vi "dt.vi"(1 "Locations Peaks":dbl[](array[numeric])) -> (0 "Tableau":dbl[](array[numeric]))   [LabVIEW 2024]
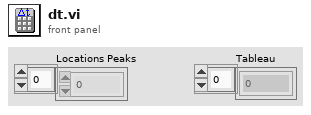
[diagram p1: front panel]
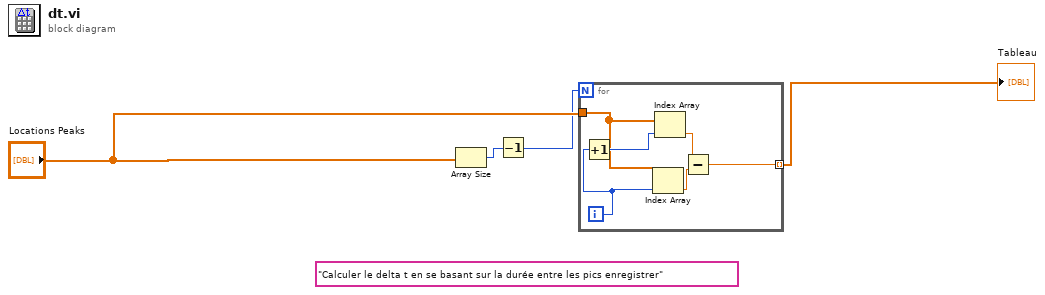
[diagram p0: block diagram]
diagram:
  (unwired) "Calculer le delta t en se basant sur la durée entre les pics enregistrer"
  n1 = Array Size(array="Locations Peaks") -> (size(s)=w1:i32)
  n2 = Decrement(x=w1) -> (x-1=w2:i32)
  n3 = for {
    N: w2 -> [_]
    tunnel: "Locations Peaks" -> [w6]
    tunnel: [w5] -> w4 mode=indexing
    i -> [w7]
    n4 = Increment(x=w7) -> (x+1=w8:i32)
    n5 = Index Array(array=w6, index=w7) -> (element=w10:dbl)
    n6 = Index Array(array=w6, index=w8) -> (element=w9:dbl)
    n7 = Subtract(x=w9, y=w10) -> (x-y=w5:dbl)
  }
  "Tableau" <- w4
